vi "Write COE file.vi"() -> ()   [LabVIEW 2015]
uses:
  Waveform parameters.ctl
panel:
  in  "Waveform parameters":T1={"Start magnitude"=1000.0, "Magnitude increment"=1000.0, "Number of pulses"=8, "Baseline length"=480, "Ramp length"=32, "Top  length"=480, "Threshold "=3000}
  in  "File Path Control":path=path "D:/github/fp/Simulation/BRAM.coe"
  out "spreadsheet string":string
  out "Step length":u32=2048
  out "Waveform length":u32
  out "Waveform Graph":dbl[](graph)
  in  "Baseline start":u16=128
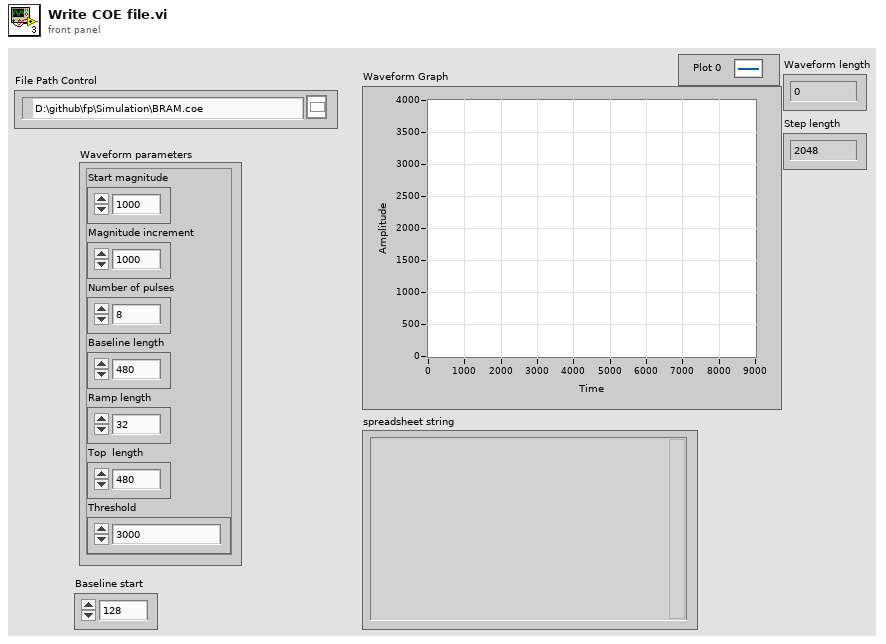
[diagram p1: front panel]
types:
  T1 = typedef "Waveform parameters.ctl" = cluster{"Start magnitude":dbl, "Magnitude increment":dbl, "Number of pulses":i32, "Baseline length":i32, "Ramp length":i32, "Top  length":i32, "Threshold ":i32}
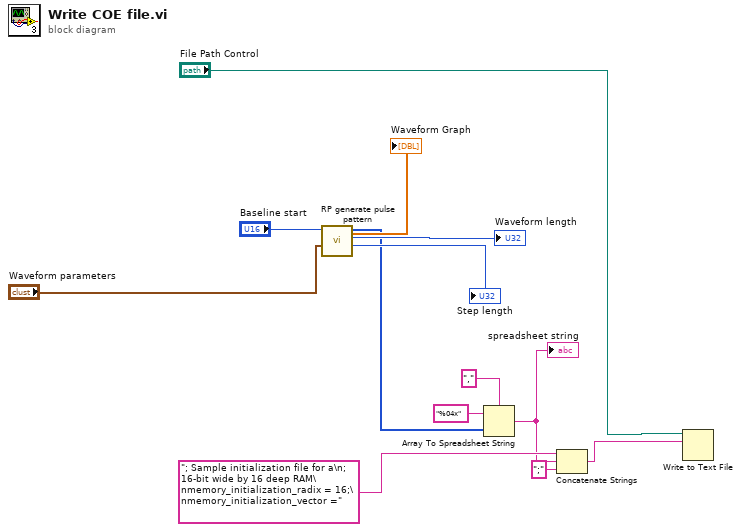
[diagram p0: block diagram]
diagram:
  n1 = call "RP generate pulse pattern.vi"("Waveform parameters"="Waveform parameters", "Baseline start"="Baseline start") -> ("Step length"=→"Step length":u32, "Waveform length"=→"Waveform length":u32, "Waveform"=w9:i16[], "Waveform Graph"=→"Waveform Graph":dbl[])  [unwired: 6 in]
  n2 = Array To Spreadsheet String(delimiter (Tab)=",", array=w9, 3:"%04x" ("format string")) -> (spreadsheet string=w4:string)
  "spreadsheet string" <- w4
  n3 = Concatenate Strings("; Sample initialization file for a\n; 16-bit wide by 16 deep RAM\nmemory_initialization_radix = 16;\nmemory_initialization_vector =" ("text"), w4, ";" ("string")) -> (w3:string)
  n4 = Write to Text File(file (use dialog)="File Path Control", text=w3) -> ()  [unwired: 2 in, 3 out]
